vi "From Control Icons to Array.vi"(1 "Control Icons":T1(array[cluster])) -> (0 "Array":refnum<class "Array.lvclass">)   [LabVIEW 2018, in "Scripts.lvlib"]
uses:
  Scripts.lvlib
  Toolkit/Data/Array/Array.lvclass
  Toolkit/Data/Map/Map.lvclass
  D:/Users/cfield/Code/Field R&D Services/Mustache/LabVIEW/trunk/src/Toolkit/Data/Abstract/Abstract.lvclass
  Toolkit/Data/Map/Support/From String Array.vi
  Toolkit/Data/Array/Support/From Data.vi
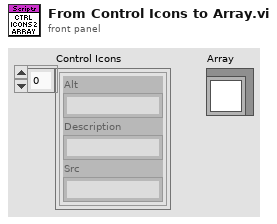
[diagram p1: front panel]
types:
  T1 = cluster{"Alt":string, "Description":string, "Src":string}[]
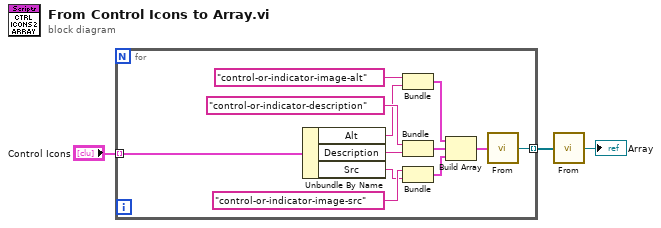
[diagram p0: block diagram]
diagram:
  n1 = for {
    tunnel: "Control Icons" -> [w15] mode=indexing
    tunnel: [w4] -> w1 mode=indexing
    n2 = Unbundle By Name(w15) -> ("Alt"=w8:string, "Description"=w7:string, "Src"=w6:string)
    n3 = Bundle("Key"="control-or-indicator-image-alt", "Alt"=w8) -> (w12:cluster{"Key":string, "Alt":string})  [unwired: 1 in]
    n4 = Bundle("Key"="control-or-indicator-description", "Description"=w7) -> (w13:cluster{"Key":string, "Description":string})  [unwired: 1 in]
    n5 = Bundle("Key"="control-or-indicator-image-src", "Src"=w6) -> (w14:cluster{"Key":string, "Src":string})  [unwired: 1 in]
    n6 = Build Array(w12, w13, w14) -> (w5:cluster{"Key":string, "Src":string}[])
    n7 = call-poly "From.vi"("Data"=w5) -> ("Map"=w4:refnum<class "Map.lvclass">)  [unwired: 1 in]
  }
  n8 = call-poly "From.vi"("Data"=w1) -> ("Array"=→"Array":refnum<class "Array.lvclass">)  [unwired: 1 in]
